vi "Write Epsilon.vi"(10 "epsilon":dbl, 11 "Equal With Epsilon Functor in":refnum<class "Equal With Epsilon Functor.lvclass">) -> (3 "Equal With Epsilon Functor out":refnum<class "Equal With Epsilon Functor.lvclass">)   [LabVIEW 2023, in "Equal With Epsilon Functor.lvclass"]
doc: "Writes the value of epsilon to use when comparing floating-point values. Pass NaN to use the epsilon value defined by the machine's CPU."
uses:
  Equal With Epsilon Functor.lvclass
  Equal With Epsilon Functor.lvclass/Equal With Epsilon Functor.ctl
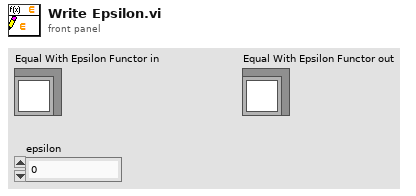
[diagram p1: front panel]
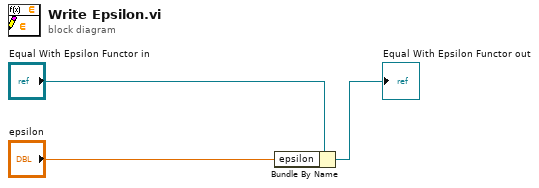
[diagram p0: block diagram]
diagram:
  n1 = Bundle By Name(cluster="Equal With Epsilon Functor in", "epsilon"="epsilon") -> (→"Equal With Epsilon Functor out":refnum<class "Equal With Epsilon Functor.lvclass">)
